vi "MouseDown.vi"(7 "Flip colors?":bool, 8 "error in":errorcluster, 10 "Coords":T5, 11 "Data in":T1={"Class"={"Ants"=refnum, "Layer"=refnum, "Templates"=refnum, "Icon"=refnum, "Glyph"=refnum, "Settings"=refnum, "Tools"=refnum}, "Ref"={"Add Layer"=refnum, "Remove Layer"=refnum, "Line Text"=[], "Body Text Spec"=refnum, "DNL_Font"=refnum, "glyph path str"=refnum, "templates path str"=refnum, "Arrow Up"=refnum, "Arrow Down"=refnum, "IE VI Ref"=refnum, "Glyphs tree"=refnum, "Templates tree"=refnum, "Layer Icon Text"=refnum, "Layer Template"=refnum, "Clipboard"=refnum, "BW icon in"=refnum, "Color icon in"=refnum, "Layer Clust"=refnum, "Body Text"=refnum, "DNL_Framework Templates"=refnum, "Search Templates"=refnum, "TextMarker"=refnum, "Tab Control"=refnum, "Search Glyphs"=refnum, "Line Color"=refnum, "DNL_Glyphs []"=refnum, "Fill Color"=refnum, "Tools"=refnum, "Glyphs tree"=refnum, "Icon"=refnum, "Preview"=refnum, "Ants"=refnum, "Terminals"=refnum, "menu reference"=refnum, "LayerNames"=[], "GlyphLoadAnimation"=refnum, "TemplateLoadAnimation"=refnum, "refreshGlyphs"=refnum, "refreshTemplates"=refnum}, "Support"={"AntsRect"={"left"=0, "top"=0, "right"=0, "bottom"=0}, "Mouse Move Coords"={"Horizontal"=0, "Vertical"=0}, "Mouse Down Coords"={"Horizontal"=0, "Vertical"=0}, "Temp Coord"={"Horizontal"=0, "Vertical"=0}, "Action"=enum."Default", "Edge Color"=4914962, "Fill Color"=16860, "Mouse Down?"=FALSE, "Draft Mode?"=FALSE, "Temp Icon"=bytes[3102], "CTRL Pressed"=FALSE, "Move Selection?"=FALSE, "AntsRect Orig"={"left"=0, "top"=0, "right"=0, "bottom"=0}, "Text"="", "TM Set?"=FALSE, "Mouse inside icon?"=FALSE, "Tool (old value)"=0, "Pencil Move Color"=0, "Swap Colors?"=FALSE, "Shift pressed?"=FALSE}}) -> (0 "error out":errorcluster, 3 "Data out":T1={"Class"={"Ants"=refnum, "Layer"=refnum, "Templates"=refnum, "Icon"=refnum, "Glyph"=refnum, "Settings"=refnum, "Tools"=refnum}, "Ref"={"Add Layer"=refnum, "Remove Layer"=refnum, "Line Text"=[], "Body Text Spec"=refnum, "DNL_Font"=refnum, "glyph path str"=refnum, "templates path str"=refnum, "Arrow Up"=refnum, "Arrow Down"=refnum, "IE VI Ref"=refnum, "Glyphs tree"=refnum, "Templates tree"=refnum, "Layer Icon Text"=refnum, "Layer Template"=refnum, "Clipboard"=refnum, "BW icon in"=refnum, "Color icon in"=refnum, "Layer Clust"=refnum, "Body Text"=refnum, "DNL_Framework Templates"=refnum, "Search Templates"=refnum, "TextMarker"=refnum, "Tab Control"=refnum, "Search Glyphs"=refnum, "Line Color"=refnum, "DNL_Glyphs []"=refnum, "Fill Color"=refnum, "Tools"=refnum, "Glyphs tree"=refnum, "Icon"=refnum, "Preview"=refnum, "Ants"=refnum, "Terminals"=refnum, "menu reference"=refnum, "LayerNames"=[], "GlyphLoadAnimation"=refnum, "TemplateLoadAnimation"=refnum, "refreshGlyphs"=refnum, "refreshTemplates"=refnum}, "Support"={"AntsRect"={"left"=0, "top"=0, "right"=0, "bottom"=0}, "Mouse Move Coords"={"Horizontal"=0, "Vertical"=0}, "Mouse Down Coords"={"Horizontal"=0, "Vertical"=0}, "Temp Coord"={"Horizontal"=0, "Vertical"=0}, "Action"=enum."Default", "Edge Color"=4914962, "Fill Color"=16860, "Mouse Down?"=FALSE, "Draft Mode?"=FALSE, "Temp Icon"=bytes[3102], "CTRL Pressed"=FALSE, "Move Selection?"=FALSE, "AntsRect Orig"={"left"=0, "top"=0, "right"=0, "bottom"=0}, "Text"="", "TM Set?"=FALSE, "Mouse inside icon?"=FALSE, "Tool (old value)"=0, "Pencil Move Color"=0, "Swap Colors?"=FALSE, "Shift pressed?"=FALSE}})   [LabVIEW 2021]
uses:
  <vilib>/Utility/miscctls.llb/LVPoint32TypeDef.ctl
  <resource>/plugins/NIIconEditor/Controls/IE Data.ctl
  <resource>/plugins/NIIconEditor/Class/Ants/Ants.lvclass
  <resource>/plugins/NIIconEditor/Class/FakedArray/FakedArray.lvclass
  <resource>/plugins/NIIconEditor/Class/Icon Library/Glyph.lvclass
  <resource>/plugins/NIIconEditor/Class/Settings/Settings.lvclass
  <resource>/plugins/NIIconEditor/Class/Tools/Tools Paint.lvclass
  <vilib>/LabVIEW Icon API/lv_icon/Classes/Icon/Icon.lvclass
  <resource>/plugins/NIIconEditor/Controls/IE Classes.ctl
  <resource>/plugins/NIIconEditor/Controls/References Cluster.ctl
  <resource>/plugins/NIIconEditor/Controls/SupportClass.ctl
  <resource>/plugins/NIIconEditor/Controls/SupportClass_Action.ctl
  <vilib>/LabVIEW Icon API/lv_icon/Controls/IEColor.ctl
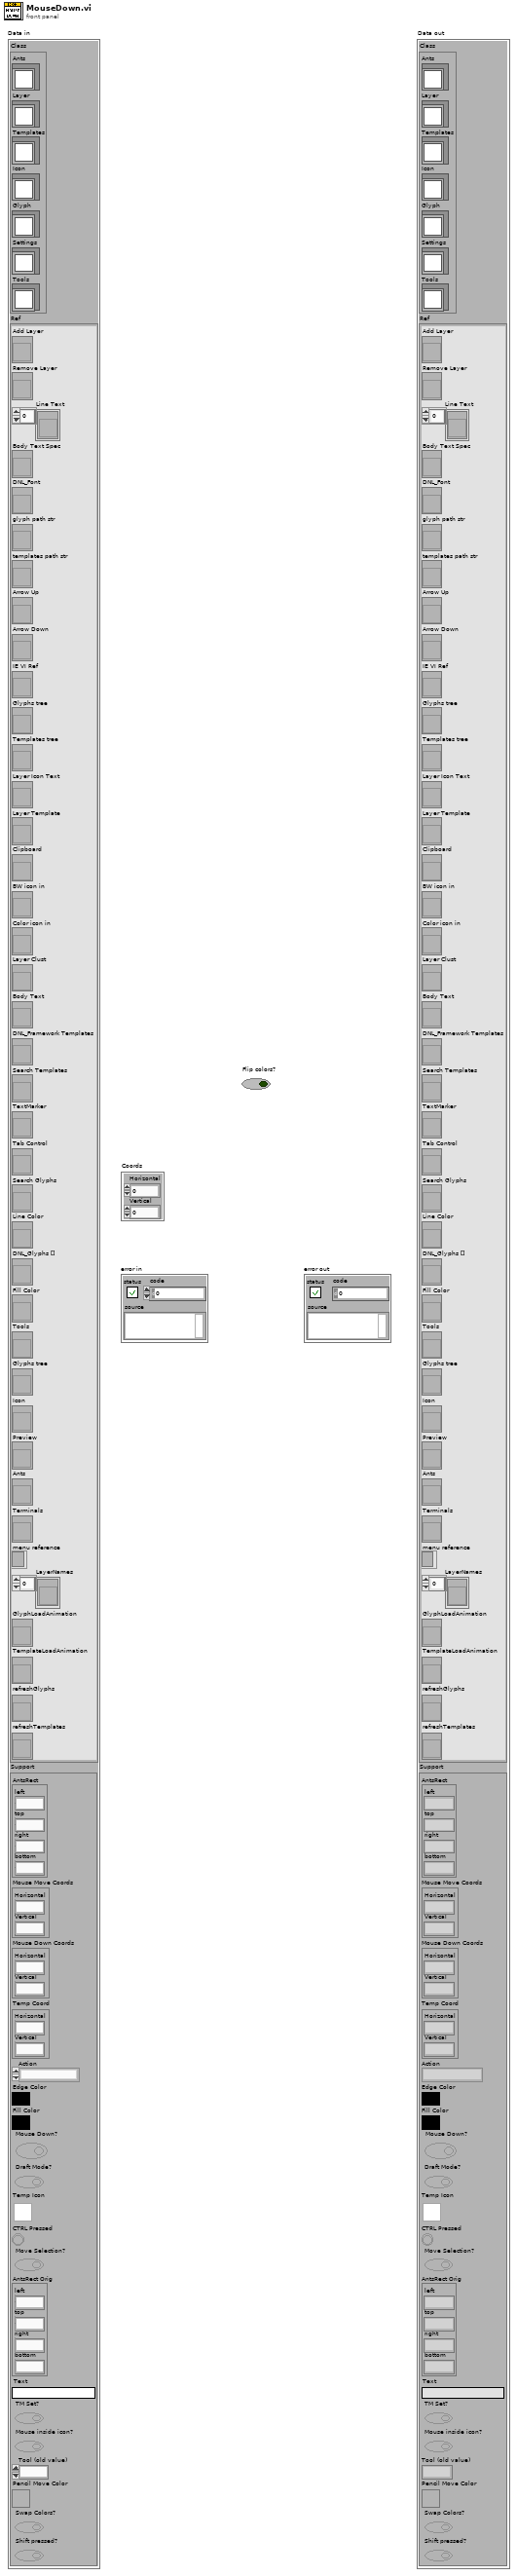
[diagram p1: front panel]
types:
  T1 = typedef "IE Data.ctl" = cluster{"Class":T2, "Ref":T3, "Support":T4}
  T2 = typedef "IE Classes.ctl" = cluster{"Ants":refnum<class "Ants.lvclass">, "Layer":refnum<class "FakedArray.lvclass">, "Templates":refnum<class "FakedArray.lvclass">, "Icon":refnum<class "Icon.lvclass">, "Glyph":refnum<class "Glyph.lvclass">, "Settings":refnum<class "Settings.lvclass">, "Tools":refnum<class "Tools Paint.lvclass">}
  T3 = typedef "References Cluster.ctl" = cluster{"Add Layer":refnum<vi>, "Remove Layer":refnum<vi>, "Line Text":refnum<vi>[], "Body Text Spec":refnum<vi>, "DNL_Font":refnum<vi>, "glyph path str":refnum<vi>, "templates path str":refnum<vi>, "Arrow Up":refnum<vi>, "Arrow Down":refnum<vi>, "IE VI Ref":refnum<vi>, "Glyphs tree":refnum<vi>, "Templates tree":refnum<vi>, "Layer Icon Text":refnum<vi>, "Layer Template":refnum<vi>, "Clipboard":refnum<vi>, "BW icon in":refnum<vi>, "Color icon in":refnum<vi>, "Layer Clust":refnum<vi>, "Body Text":refnum<vi>, "DNL_Framework Templates":refnum<vi>, "Search Templates":refnum<vi>, "TextMarker":refnum<vi>, "Tab Control":refnum<vi>, "Search Glyphs":refnum<vi>, "Line Color":refnum<vi>, "DNL_Glyphs []":refnum<vi>, "Fill Color":refnum<vi>, "Tools":refnum<vi>, "Glyphs tree":refnum<vi>, "Icon":refnum<vi>, "Preview":refnum<vi>, "Ants":refnum<vi>, "Terminals":refnum<vi>, "menu reference":refnum<k9>, "LayerNames":refnum<vi>[], "GlyphLoadAnimation":refnum<vi>, "TemplateLoadAnimation":refnum<vi>, "refreshGlyphs":refnum<vi>, "refreshTemplates":refnum<vi>}
  T4 = typedef "SupportClass.ctl" = cluster{"AntsRect":cluster{"left":i16, "top":i16, "right":i16, "bottom":i16}, "Mouse Move Coords":T5, "Mouse Down Coords":T5, "Temp Coord":T5, "Action":T6, "Edge Color":T7, "Fill Color":T7, "Mouse Down?":bool, "Draft Mode?":bool, "Temp Icon":picture, "CTRL Pressed":bool, "Move Selection?":bool, "AntsRect Orig":cluster{"left":i16, "top":i16, "right":i16, "bottom":i16}, "Text":string, "TM Set?":bool, "Mouse inside icon?":bool, "Tool (old value)":u32, "Pencil Move Color":u32, "Swap Colors?":bool, "Shift pressed?":bool}
  T5 = typedef "LVPoint32TypeDef.ctl" = cluster{"Horizontal":i32, "Vertical":i32}
  T6 = typedef "SupportClass_Action.ctl" = enum16{"Default", "Move Selection", "Glyph Library", "Tool"}
  T7 = typedef "IEColor.ctl" = u32
  T8 = cluster{"left":i16, "top":i16, "right":i16, "bottom":i16}
  T9 = typedef "Tools.ctl" = enum32{"Pencil", "Line", "Dropper", "Fill", "Rectangle", "Filled Rectangle", "Ellipse", "Filled Ellipse", "Eraser", "Text", "Select", "Move"}
  T10 = cluster{"Horizontal":i32, "Vertical":i32, "Vertical 2":i32, "Vertical 3":i32}
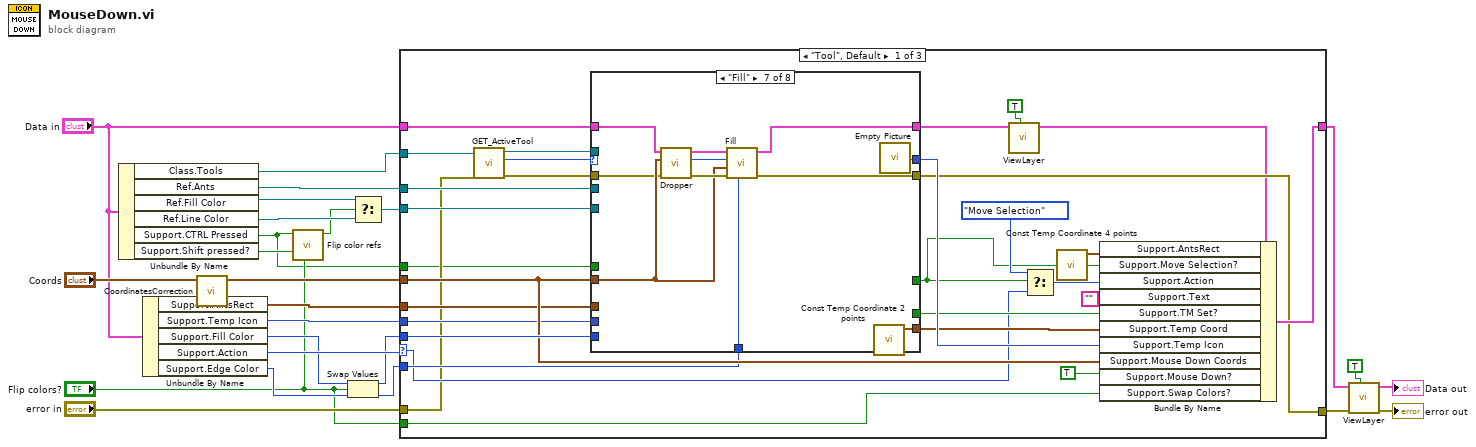
[diagram p0: block diagram]
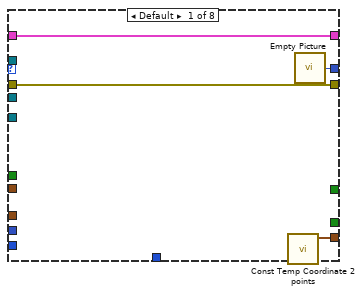
[diagram p2: hidden frame]
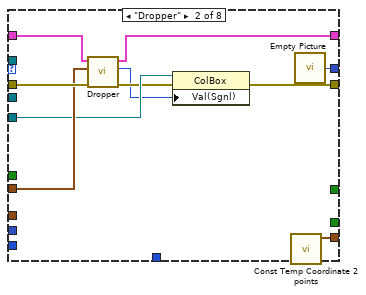
[diagram p3: hidden frame]
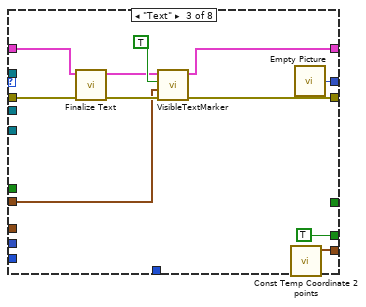
[diagram p4: hidden frame]
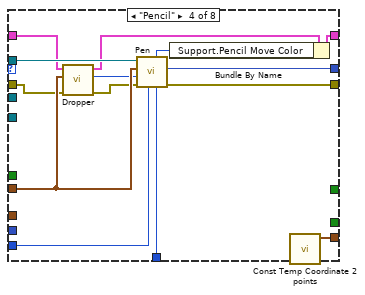
[diagram p5: hidden frame]
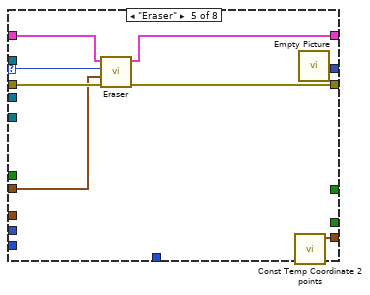
[diagram p6: hidden frame]
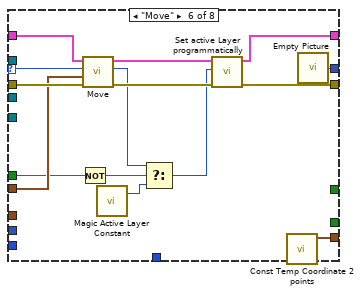
[diagram p7: hidden frame]
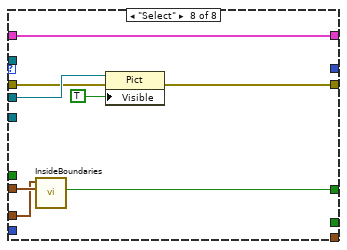
[diagram p8: hidden frame]
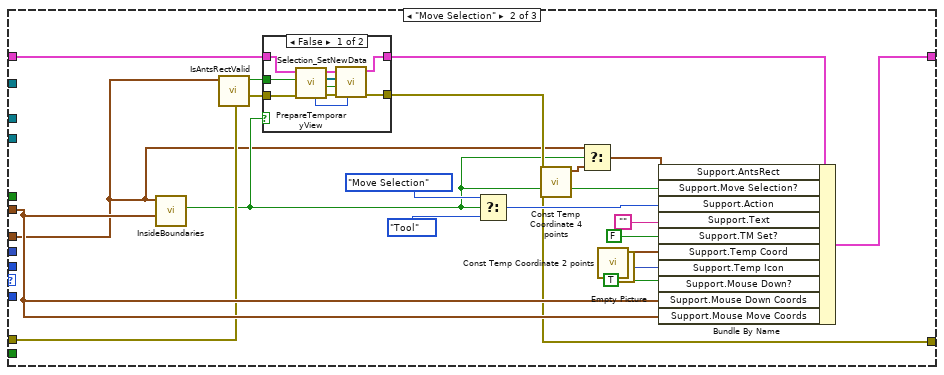
[diagram p9: hidden frame]
diagram:
  n1 = Unbundle By Name("Data in") -> ("Class.Tools"=w19:refnum<class "Tools Paint.lvclass">, "Ref.Ants"=w21:refnum<vi>, "Ref.Fill Color"=w6:refnum<vi>, "Ref.Line Color"=w5:refnum<vi>, "Support.CTRL Pressed"=w1:bool, "Support.Shift pressed?"=w2:bool)
  n2 = Unbundle By Name("Data in") -> ("Support.AntsRect"=w20:T8, "Support.Temp Icon"=w22:picture, "Support.Fill Color"=w9:T7, "Support.Action"=w24:T6, "Support.Edge Color"=w11:T7)
  n3 = call <resource>:"CoordinatesCorrection.vi"("Coordinates In"="Coords") -> ("Corrected Out"=w25:T5)  [unwired: 10 out]
  n4 = call <resource>:"Flip color refs.vi"("Flip colors?"="Flip colors?", "Shift pressed"=w2, "CTRL pressed"=w1) -> ("Flip?"=w3:bool)  [unwired: 8 out]
  n5 = Swap Values(12:w9, 13:"Flip colors?", 14:w11) -> (1:w8:T7, 3:w10:T7)
  n6 = Select(t=w6, s=w3, f=w5) -> (s? t:f=w7:refnum<vi>)
  n7 = case shown="\"Tool\", Default" w24 {
    selector: w24 -> [w40 _ _]
    tunnel: [w48 w143 w169] -> w15
    tunnel: w25 -> [w51 w146 _]
    tunnel: "error in" -> [w33 w144 w169]
    tunnel: [w49 w151 w168] -> w12
    tunnel: w8 -> [w52 _ _]
    tunnel: w10 -> [w47 _ _]
    tunnel: w22 -> [w44 _ _]
    tunnel: w21 -> [w43 _ _]
    tunnel: w20 -> [w42 w139 _]
    tunnel: w7 -> [w36 _ _]
    tunnel: w19 -> [w34 _ _]
    tunnel: "Data in" -> [w32 w142 w168]
    tunnel: "Flip colors?" -> [w31 _ _]
    tunnel: w1 -> [w29 _ _]
    frame "Tool", Default {
      n8 = call-dynamic "GET_ActiveTool.vi"("error in (no error)"=w33, "Tools Paint.lvclass in"=w34) -> ("error out"=w54:errorcluster, "Radio Buttons"=w55:T9, "Tools Paint.lvclass out"=w37:refnum<class "Tools Paint.lvclass">)  [unwired: 7 out]
      n9 = case shown="\"Fill\"" w55 {
        selector: w55 -> [_ _ _ _ w98 w114 _ _]
        tunnel: w54 -> [w59 w68 w76 w89 w101 w116 w123 w130]
        tunnel: w51 -> [_ w66 w70 w90 w99 w115 w124 w133]
        tunnel: w52 -> [_ _ _ w81 _ _ _ _]
        tunnel: [w58 w69 w77 w94 w102 w117 w127 _] -> w50
        tunnel: [w59 w67 w79 w93 w100 w111 w126 w134] -> w48
        tunnel: w47 -> [_ _ _ w82 _ _ w118 _]
        tunnel: [w57 w65 w80 w92 w97 w113 w128 _] -> w46
        tunnel: [_ _ TRUE ("Mouse Down?") _ _ _ _ _] -> w45
        tunnel: w44 -> [_ _ _ _ _ _ _ _]
        tunnel: w43 -> [_ _ _ _ _ _ _ w136]
        tunnel: w42 -> [_ _ _ _ _ _ _ w132]
        tunnel: [_ _ _ _ _ _ _ w131] -> w35
        tunnel: w37 -> [_ _ _ w91 _ _ _ _]
        tunnel: w36 -> [_ w64 _ _ _ _ _ _]
        tunnel: w32 -> [w56 w63 w74 w86 w96 w110 w121 w129]
        tunnel: [w56 w62 w71 w84 w95 w108 w119 w129] -> w27
        tunnel: w29 -> [_ _ _ _ _ w107 _ _]
        frame Default {
          n10 = call <resource>:"Const Temp Coordinate 2 points.vi"() -> ("Const Temp Coordinate"=w57:T5)  [unwired: 11 out]
          n11 = call "Empty Picture"() -> ("empty picture"=w58:picture)
        }
        frame "Dropper" {
          n12 = call <resource>:"Dropper.vi"("error in (no error)"=w68, "point(x,y)"=w66, "Data in"=w63) -> ("error out"=w61:errorcluster, "Color"=w60:u32, "Data out"=w62:T1)  [unwired: 1 in, 5 out]
          n13 = property on="Property Node" class="ColBox"(reference=w64, error in=w61, "Val(Sgnl)"=w60) -> (error out=w67:errorcluster)  [unwired: 1 out]
          n14 = call <resource>:"Const Temp Coordinate 2 points.vi"() -> ("Const Temp Coordinate"=w65:T5)  [unwired: 11 out]
          n15 = call "Empty Picture"() -> ("empty picture"=w69:picture)
        }
        frame "Text" {
          n16 = call <resource>:"Finalize Text.vi"("error in (no error)"=w76, "Data in"=w74) -> ("error out"=w75:errorcluster, "Data out"=w72:T1)  [unwired: 8 out]
          n17 = call <resource>:"VisibleTextMarker.vi"("error in (no error)"=w75, "Position"=w70, "Visible"=TRUE, "Data in"=w72) -> ("error out"=w79:errorcluster, "Data out"=w71:T1)  [unwired: 6 out]
          n18 = call <resource>:"Const Temp Coordinate 2 points.vi"() -> ("Const Temp Coordinate"=w80:T5)  [unwired: 11 out]
          n19 = call "Empty Picture"() -> ("empty picture"=w77:picture)
        }
        frame "Pencil" {
          n20 = call <resource>:"Dropper.vi"("error in (no error)"=w89, "point(x,y)"=w90, "Data in"=w86) -> ("error out"=w88:errorcluster, "Color"=w87:u32, "Data out"=w85:T1)  [unwired: 6 out]
          n21 = call-dynamic "Pen.vi"("Edge color"=w82, "Fill color"=w81, "error in (no error)"=w88, "Current color (T)"=w87, "point(x,y)"=w90, "Tools Paint in"=w91) -> ("error out"=w93:errorcluster, "new picture"=w94:picture, "Current line color"=w83:u32)  [unwired: 3 out]
          n22 = Bundle By Name(cluster=w85, "Support.Pencil Move Color"=w83) -> (w84:T1)
          n23 = call <resource>:"Const Temp Coordinate 2 points.vi"() -> ("Const Temp Coordinate"=w92:T5)  [unwired: 11 out]
        }
        frame "Eraser" {
          n24 = call <resource>:"Eraser.vi"("error in (no error)"=w101, "point(x,y)"=w99, "Radio Buttons"=w98, "Data in"=w96) -> ("error out"=w100:errorcluster, "Data out"=w95:T1)  [unwired: 1 in, 5 out]
          n25 = call <resource>:"Const Temp Coordinate 2 points.vi"() -> ("Const Temp Coordinate"=w97:T5)  [unwired: 11 out]
          n26 = call "Empty Picture"() -> ("empty picture"=w102:picture)
        }
        frame "Move" {
          n27 = Not(x=w107) -> (.not. x?=w106:bool)
          n28 = call <resource>:"Move.vi"("error in (no error)"=w116, "point(x,y)"=w115, "Tools"=w114, "Data in"=w110) -> ("error out"=w112:errorcluster, "Active Layer"=w105:i32, "Data out"=w109:T1)  [unwired: 1 in, 4 out]
          n29 = call <resource>:"Magic Active Layer Constant.vi"() -> ("Magic Constant"=w104:i32)  [unwired: 19 out]
          n30 = Select(t=w105, s=w106, f=w104) -> (s? t:f=w103:i32)
          n31 = call <resource>:"Set active Layer programmatically.vi"("error in"=w112, "Active Layer"=w103, "Data in"=w109) -> ("error out"=w111:errorcluster, "Data out"=w108:T1)  [unwired: 1 in, 6 out]
          n32 = call <resource>:"Const Temp Coordinate 2 points.vi"() -> ("Const Temp Coordinate"=w113:T5)  [unwired: 11 out]
          n33 = call "Empty Picture"() -> ("empty picture"=w117:picture)
        }
        frame "Fill" {
          n34 = call <resource>:"Dropper.vi"("error in (no error)"=w123, "point(x,y)"=w124, "Data in"=w121) -> ("error out"=w125:errorcluster, "Color"=w122:u32, "Data out"=w120:T1)  [unwired: 6 out]
          n35 = call <resource>:"Fill.vi"("Color"=w118, "error in (no error)"=w125, "point(x,y)"=w124, "Ref Color"=w122, "Data in"=w120) -> ("error out"=w126:errorcluster, "Data out"=w119:T1)  [unwired: 1 in, 4 out]
          n36 = call <resource>:"Const Temp Coordinate 2 points.vi"() -> ("Const Temp Coordinate"=w128:T5)  [unwired: 11 out]
          n37 = call "Empty Picture"() -> ("empty picture"=w127:picture)
        }
        frame "Select" {
          n38 = call <resource>:"InsideBoundaries.vi"("Mouse Move Coords"=w133, "AntsRect"=w132) -> ("Inside?"=w131:bool)  [unwired: 9 out]
          n39 = property class="Pict"(reference=w136, error in=w130, "Visible"=TRUE) -> (error out=w134:errorcluster)  [unwired: 1 out]
        }
      }
      n40 = call <resource>:"ViewLayer.vi"("Add to Undo?"=TRUE, "Data in"=w27) -> ("Data out"=w26:T1)  [unwired: 2 in, 7 out]
      n41 = Select(t=SupportClass_Action."Move Selection", s=w35, f=w40) -> (s? t:f=w38:T6)
      n42 = call <resource>:"Const Temp Coordinate 4 points.vi"() -> ("Const Temp Coordinate"=w30:T10)  [unwired: 11 out]
      n43 = Bundle By Name(cluster=w26, "Support.AntsRect"=w30, "Support.Move Selection?"=w35, "Support.Action"=w38, "Support.Text"="", "Support.TM Set?"=w45, "Support.Temp Coord"=w46, "Support.Temp Icon"=w50, "Support.Mouse Down Coords"=w51, "Support.Mouse Down?"=TRUE ("Mouse Down?"), "Support.Swap Colors?"=w31) -> (w49:T1)
    }
    frame "Move Selection" {
      n44 = call <resource>:"InsideBoundaries.vi"("Mouse Move Coords"=w146, "AntsRect"=w139) -> ("Inside?"=w140:bool)  [unwired: 9 out]
      n45 = call <resource>:"IsAntsRectValid.vi"("AntsRect"=w139) -> ("Valid?"=w145:bool)  [unwired: 10 out]
      n46 = case shown="False" w140 {
        tunnel: w145 -> [w162 _]
        tunnel: w144 -> [w161 w167]
        tunnel: [w160 w167] -> w143
        tunnel: w142 -> [w158 w166]
        tunnel: [w156 w166] -> w141
        frame False {
          n47 = call <resource>:"PrepareTemporaryView.vi"("error in (no error)"=w161, "Valid Selection?"=w162, "Data in"=w158) -> ("error out"=w159:errorcluster, "Highlighted?"=w164:bool, "All Layers out"=w165:refnum<class "Layer.lvclass">[], "Data out"=w157:T1, "#Active Layer"=w163:i32)  [unwired: 2 in, 2 out]
          n48 = call <resource>:"Selection_SetNewData.vi"("#Active Layer"=w163, "error in"=w159, "Highlighted?"=w164, "All Layers In"=w165, "Data in"=w157) -> ("error out"=w160:errorcluster, "Data out"=w156:T1)  [unwired: 1 in, 3 out]
        }
        frame True {
        }
      }
      n49 = Select(t=SupportClass_Action."Move Selection", s=w140, f=SupportClass_Action."Tool") -> (s? t:f=w150:T6)
      n50 = call <resource>:"Const Temp Coordinate 4 points.vi"() -> ("Const Temp Coordinate"=w138:T10)  [unwired: 11 out]
      n51 = Select(t=w139, s=w140, f=w138) -> (s? t:f=w137:T10)
      n52 = call <resource>:"Const Temp Coordinate 2 points.vi"() -> ("Const Temp Coordinate"=w149:T5)  [unwired: 11 out]
      n53 = call "Empty Picture"() -> ("empty picture"=w148:picture)
      n54 = Bundle By Name(cluster=w141, "Support.AntsRect"=w137, "Support.Move Selection?"=w140, "Support.Action"=w150, "Support.Text"="", "Support.TM Set?"=FALSE ("TM Set?"), "Support.Temp Coord"=w149, "Support.Temp Icon"=w148, "Support.Mouse Down?"=TRUE ("Mouse Down?"), "Support.Mouse Down Coords"=w146, "Support.Mouse Move Coords"=w146) -> (w151:T1)
    }
    frame "Glyph Library" {
    }
  }
  n55 = call <resource>:"ViewLayer.vi"("Add to Undo?"=TRUE, "error in (no error)"=w15, "Data in"=w12) -> ("error out"=→"error out":errorcluster, "Data out"=→"Data out":T1)  [unwired: 1 in, 6 out]
